vi "acquire_error.vi"(8 "error in (no error)":errorcluster) -> (0 "error out":errorcluster)   [LabVIEW 2020]
uses:
  FGVs/FGVstates.ctl
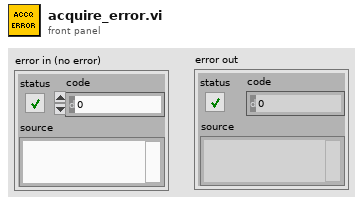
[diagram p1: front panel]
types:
  T1 = typedef "FGVstates.ctl" = enum16{"Init", "Set", "Get", "De-Init"}
  T2 = typedef "data_exchange_fgv.ctl" = cluster{"queue states":refnum<queue>, "audio data":refnum<queue>, "error queue":refnum<queue>}
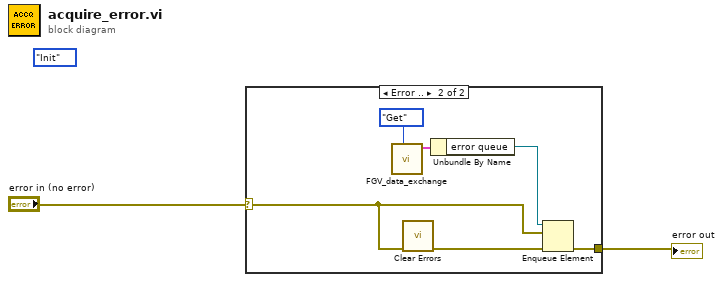
[diagram p0: block diagram]
diagram:
  (unwired) FGVstates."Init" ("FGV states")
  n1 = case shown="Error .." "error in (no error)" {
    selector: "error in (no error)" -> [w3 w4]
    tunnel: [w3 w5] -> w1
    frame No Error {
    }
    frame Error {
      n2 = call "FGV_data_exchange.vi"("FGV states"=FGVstates."Get") -> ("main_cycle_queue"=w8:T2)  [unwired: 9 in, 1 out]
      n3 = call <vilib>:"Clear Errors.vi"("error in (no error)"=w4) -> ("error out"=w7:errorcluster)  [unwired: 5 in, 1 out]
      n4 = Unbundle By Name(w8) -> ("error queue"=w6:refnum<queue>)
      n5 = Enqueue Element(queue=w6, element=w4, error in (no error)=w7) -> (error out=w5:errorcluster)  [unwired: 1 in, 2 out]
    }
  }
  "error out" <- w1
